vi "Hidden Numbers Single Pole Differentiator.vi"(1 "18b (s-fxp-1) Input (A)":fxp<+/-,18,1> format="%.18g", 2 "N":fxp<+,6,6>) -> (0 "18b (s-fxp-1) out":fxp<+/-,18,1> format="%.18g")   [LabVIEW 2010]
panel:
  out "(Y/z)(1-2^-N)+(A-A/z)":fxp<+/-,64,47> format="%.32g"
  out "(A-A/z)+Y/z":fxp<+/-,64,47> format="%.32g"
  out "Input (A) sub zero":fxp<+/-,18,1> format="%.18g"
  # "64b (s-fxp-47) internal representation"
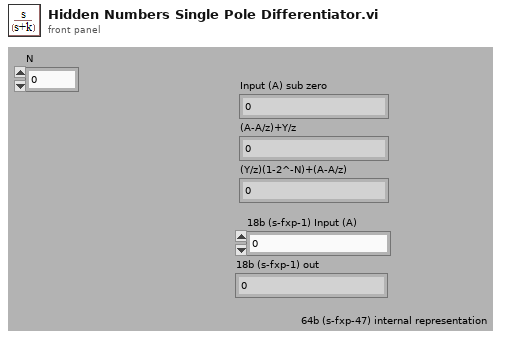
[diagram p1: front panel]
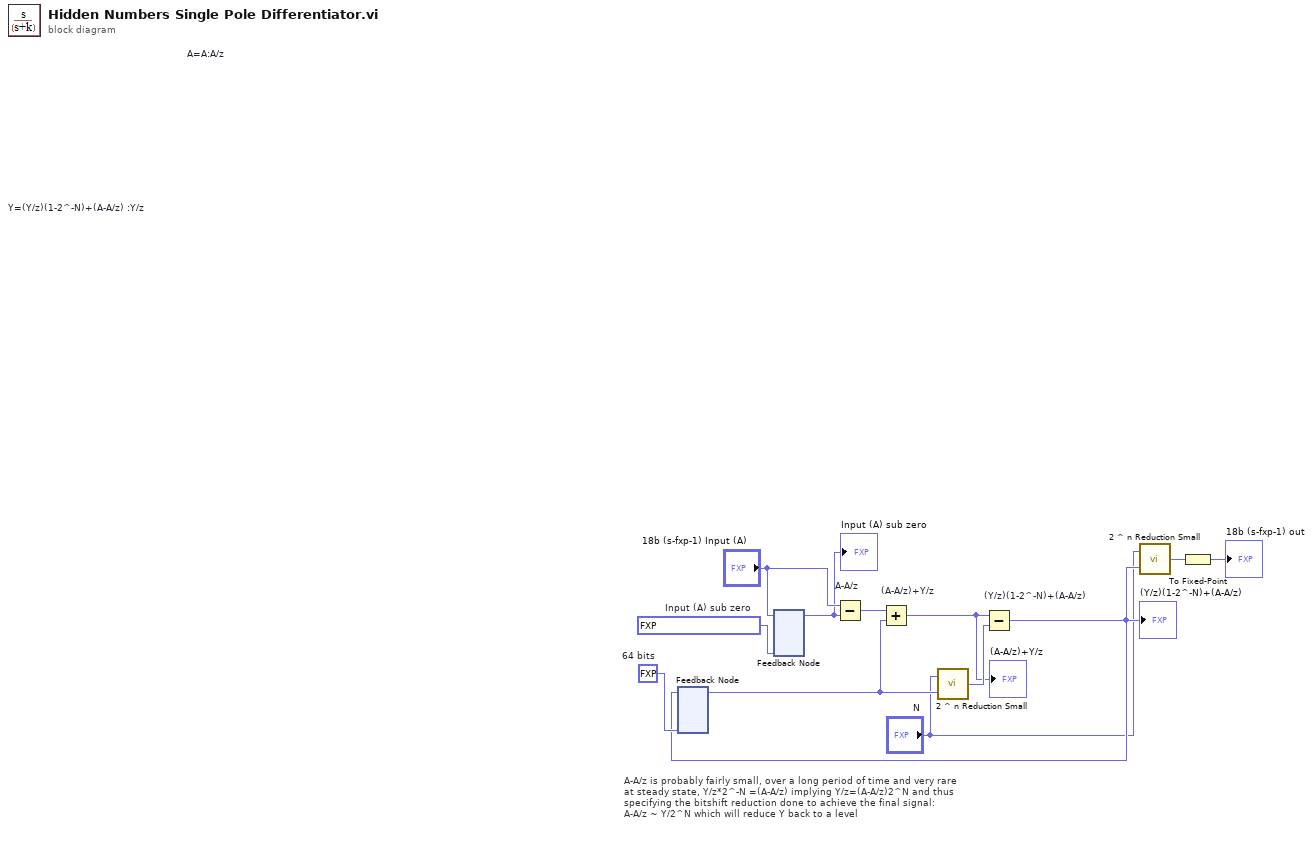
[diagram p0: block diagram]
diagram:
  w5 = fxp<+/-,18,1> 0.0  # Input (A) sub zero
  w10 = fxp<+/-,64,47> 0.0  # 64 bits
  # "A-A/z is probably fairly small, over a long period of time and very rare\nat steady state, Y/z*2^-N =(A-A/z) implying Y/z=(A-A/z)2^N and thus \nspecifying the bitshift reduction done to achieve the final signal:\nA-A/z ~ Y/2^N which will reduce Y back to a level"
  n1 = feedback #1 "Y=(Y/z)(1-2^-N)+(A-A/z) :Y/z"(w10) -> (w8:fxp<+/-,64,47>)
  n2 = feedback-in #2("18b (s-fxp-1) Input (A)") -> ()
  n3 = feedback #2 "A=A:A/z"(w5) -> (w11:fxp<+/-,18,1>)
  "Input (A) sub zero" <- w11
  n4 = Subtract "A-A/z"(x="18b (s-fxp-1) Input (A)", y=w11) -> (x-y=w9:fxp<+/-,18,1>)
  n5 = Add "(A-A/z)+Y/z"(x=w9, y=w8) -> (x+y=w6:fxp<+/-,64,47>)
  "(A-A/z)+Y/z" <- w6
  n6 = call "2 ^ n Reduction Small.vi"("64b (s-fxp-47) in"=w8, "N"="N") -> ("64b (s-fxp-47) out"=w7:fxp<+/-,64,47>)
  n7 = Subtract "(Y/z)(1-2^-N)+(A-A/z)"(x=w6, y=w7) -> (x-y=w4:fxp<+/-,64,47>)
  "(Y/z)(1-2^-N)+(A-A/z)" <- w4
  n8 = feedback-in #1(w4) -> ()
  n9 = call "2 ^ n Reduction Small.vi"("64b (s-fxp-47) in"=w4, "N"="N") -> ("64b (s-fxp-47) out"=w2:fxp<+/-,64,47>)
  n10 = To Fixed-Point(number=w2) -> (fixed-point=→"18b (s-fxp-1) out":fxp<+/-,18,1>)  [unwired: 1 in]
